vi "Run IntClk Device.vi"(0 "Dig out task":refnum<k21>, 2 "Oversample clock rate":dbl=1000.0 format="%0.2f", 5 "Dig in task":refnum<k21>, 9 "Digital waveform":digitalwaveform(waveform)={"t0"=timestamp(0 s since 1904-01-01), "dt"=0.0, "Y"={"transitions"=[], "data"=[]}, "error"={"status"=FALSE, "code"=37421928, "source"=""}}, 11 "error in (no error)":errorcluster) -> (4 "Dig out task out":refnum<k21>, 6 "Dig in task out":refnum<k21>, 10 "Input ch data":digitalwaveform(waveform)={"t0"=timestamp(0 s since 1904-01-01), "dt"=1.0, "Y"={"transitions"=[], "data"=[]}}, 15 "error out":errorcluster)   [LabVIEW 2016, in "SPIVI.lvlib"]
uses:
  <vilib>/DAQmx/write.llb/DAQmx Write (Digital Wfm 1Chan NSamp).vi
  <vilib>/DAQmx/read.llb/DAQmx Read (Digital Wfm 1Chan NSamp).vi
  <vilib>/Waveform/DWDTOps.llb/DWDT Digital Size.vi
  <vilib>/DAQmx/configure/timing.llb/DAQmx Timing (Sample Clock).vi
  <vilib>/Waveform/DWDTOps.llb/DWDT Uncompress Digital.vi
  <vilib>/DAQmx/miscellaneous.llb/DAQmx Fill In Error Info.vi
  SPIVI.lvlib
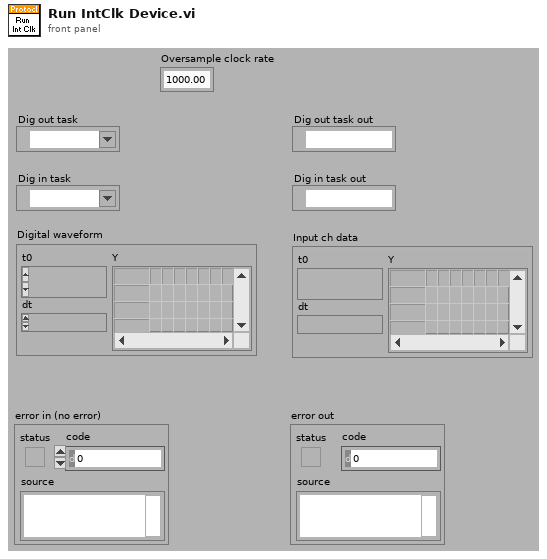
[diagram p1: front panel]
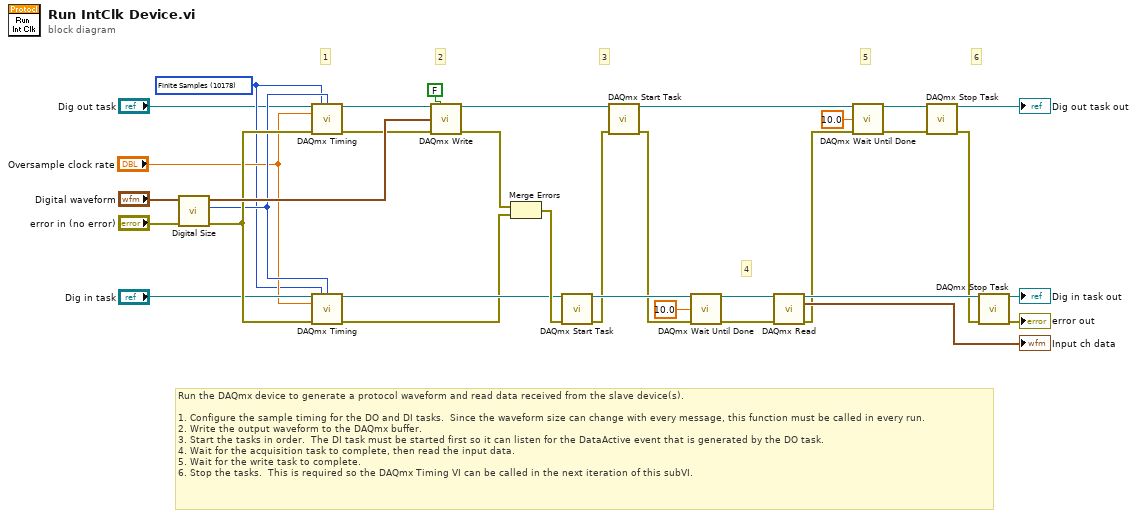
[diagram p0: block diagram]
diagram:
  w17 = 10178 items=["Finite Samples"=10178, "Continuous Samples"=10123] ("sample mode")
  # "5"
  # "Run the DAQmx device to generate a protocol waveform and read data received from the slave device(s).\n\n1. Configure the sample timing for the DO and DI tasks.  Since the waveform size can change with every message, this function must be called in every run.\n2. Write the output waveform to the DAQmx buffer.\n3. Start the tasks in order.  The DI task must be started first so it can listen for the DataActive event that is generated by the DO task.\n4. Wait for the acquisition task to complete, then read the input data.\n5. Wait for the write task to complete.\n6. Stop the tasks.  This is required so the DAQmx Timing VI can be called in the next iteration of this subVI."
  # "6"
  # "4"
  # "3"
  # "2"
  # "1"
  n1 = call-poly <vilib>:"Digital Size.vi"("error in (no error)"="error in (no error)", "digital waveform in"="Digital waveform") -> ("error out"=w21:errorcluster, "number of samples"=w20:i32, "digital waveform out"=w26:digitalwaveform)  [unwired: 7 out]
  n2 = call-poly <vilib>:"DAQmx Timing.vi"("task/channels in"="Dig out task", "sample mode"=w17, "samples per channel"=w20, "rate"="Oversample clock rate", "error in"=w21) -> ("task out"=w8:refnum<k21>, "error out"=w9:errorcluster)  [unwired: 2 in, 7 out]
  n3 = call-poly <vilib>:"DAQmx Timing.vi"("task/channels in"="Dig in task", "sample mode"=w17, "samples per channel"=w20, "rate"="Oversample clock rate", "error in"=w21) -> ("task out"=w7:refnum<k21>, "error out"=w6:errorcluster)  [unwired: 2 in, 7 out]
  n4 = call-poly <vilib>:"DAQmx Write.vi"("task/channels in"=w8, "auto start"=FALSE, "data"=w26, "error in"=w9) -> ("task out"=w34:refnum<k21>, "error out"=w28:errorcluster)  [unwired: 10 out]
  n5 = Merge Errors(w28, w6) -> (w13:errorcluster)
  n6 = call <vilib>:"DAQmx Start Task.vi"("task/channels in"=w7, "error in"=w13) -> ("task out"=w25:refnum<k21>, "error out"=w12:errorcluster)  [unwired: 12 out]
  n7 = call <vilib>:"DAQmx Start Task.vi"("task/channels in"=w34, "error in"=w12) -> ("task out"=w5:refnum<k21>, "error out"=w11:errorcluster)  [unwired: 12 out]
  n8 = call <vilib>:"DAQmx Wait Until Done.vi"("task/channels in"=w25, "timeout (sec)"=10.0, "error in"=w11) -> ("task out"=w23:refnum<k21>, "error out"=w24:errorcluster)  [unwired: 11 out]
  n9 = call-poly <vilib>:"DAQmx Read.vi"("task/channels in"=w23, "error in"=w24) -> ("task out"=w32:refnum<k21>, "data"=→"Input ch data":digitalwaveform, "error out"=w3:errorcluster)  [unwired: 2 in, 9 out]
  n10 = call <vilib>:"DAQmx Wait Until Done.vi"("task/channels in"=w5, "timeout (sec)"=10.0, "error in"=w3) -> ("task out"=w4:refnum<k21>, "error out"=w2:errorcluster)  [unwired: 11 out]
  n11 = call <vilib>:"DAQmx Stop Task.vi"("task/channels in"=w4, "error in"=w2) -> ("task out"=→"Dig out task out":refnum<k21>, "error out"=w31:errorcluster)  [unwired: 12 out]
  n12 = call <vilib>:"DAQmx Stop Task.vi"("task/channels in"=w32, "error in"=w31) -> ("task out"=→"Dig in task out":refnum<k21>, "error out"=→"error out":errorcluster)  [unwired: 12 out]
